vi "Convert Dependency Array (VIPM to NIPM).vi"(8 "error in (no error)":errorcluster, 9 "LabVIEW version in":string, 11 "VIPM dependency string array":string[](array[string])) -> (0 "error out":errorcluster, 1 "LabVIEW version out":string, 3 "NIPM dependency string array":string[](array[string]))   [LabVIEW 2014, in "vipm-to-nipm-package-converter.lvlib"]
doc: "Converts the VIPM package's Display Name to a LabVIEW-version specific NIPM Package Display Name. For example, \"oglib_string>=4.1.0.12\" and \"18.0\" converts to \"oglib-string-lv2018-32-bit (>= 4.1.9.12)\".\n\nINPUT(S):\n<b>LabVIEW version</b>: Specifies the LabVIEW version for the NIPM package to support (\"14.0\", \"14.0 (64-bit)\", \"18.0\", \"18.0 (64-bit)\", etc)"
uses:
  vipm-to-nipm-package-converter.lvlib
  <vilib>/regexp/Match Regular Expression.xnode
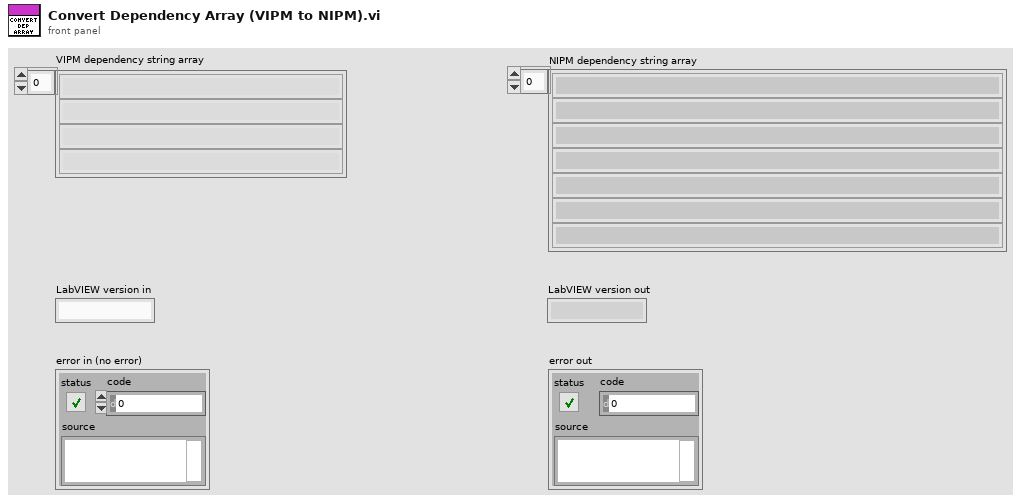
[diagram p1: front panel]
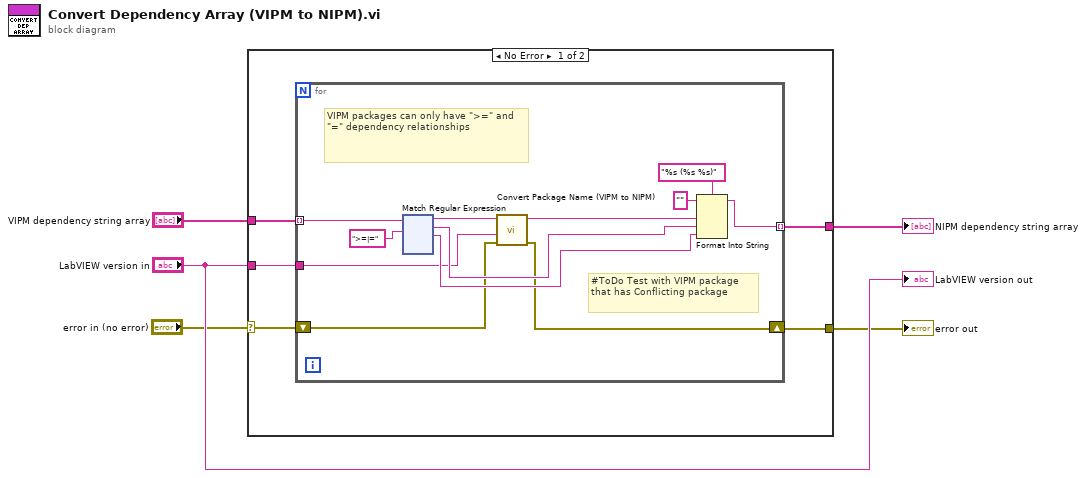
[diagram p0: block diagram]
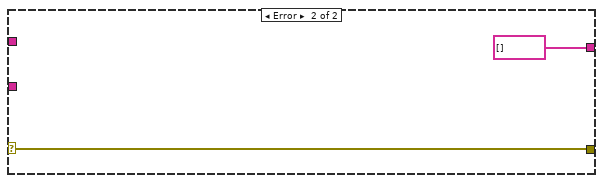
[diagram p2: hidden frame]
diagram:
  n1 = case shown="No Error" "error in (no error)" {
    selector: "error in (no error)" -> [w6 w138]
    tunnel: "LabVIEW version in" -> [w10 _]
    tunnel: [w9 string[] []] -> w4
    tunnel: [w8 w138] -> w3
    tunnel: "VIPM dependency string array" -> [w7 _]
    frame No Error {
      n2 = for {
        tunnel: w7 -> [w16] mode=indexing
        tunnel: w10 -> [w11]
        tunnel: [w17] -> w9 mode=indexing
        shift-right: [w14] -> w8
        shift-left: w6 -> [w15]
        # "#ToDo Test with VIPM package that has Conflicting package"
        # "VIPM packages can only have \">=\" and \"=\" dependency relationships"
        n3 = xnode "Match Regular Expression"("input string"=w16, "regular expression"=">=|=") -> ("before match"=w21:string, "whole match"=w19:string, "after match"=w18:string)  [unwired: 4 in, 2 out]
        n4 = call "Convert Package Name (VIPM to NIPM).vi"("error in (no error)"=w15, "LabVIEW version in"=w11, "VIPM Package Name"=w21) -> ("error out"=w14:errorcluster, "NIPM Package Name"=w20:string)  [unwired: 6 in, 1 out]
        n5 = Format Into String(format string="%s (%s %s)" ("string"), initial string="", w20, w19, w18) -> (resulting string=w17:string)  [unwired: 1 in, 1 out]
      }
    }
    frame Error {
    }
  }
  "NIPM dependency string array" <- w4
  "error out" <- w3
  "LabVIEW version out" <- "LabVIEW version in"
